vi "SubVI_Files_to_epochs_rev2.vi"(6 "Ch_sel":i32[](array[numeric])=[0, 1, 1, 1, 0], 8 "error in (no error)":errorcluster, 9 "Restrict?":bool, 11 "folder names":string[](array[string])) -> (0 "error out":errorcluster, 1 "Number of Trials":i32, 2 "Rest Epochs":dbl[][](array[numeric]), 3 "Go Epochs":dbl[][](array[numeric]))   [LabVIEW 2020]
uses:
  <vilib>/Analysis/baseanly.llb/Mean (DBL).vi
  <vilib>/Analysis/NI_AALBase.lvlib
panel:
  out "Trial number":i32
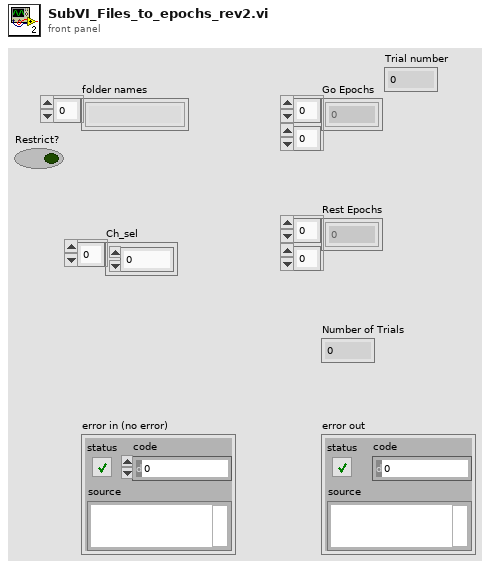
[diagram p1: front panel]
types:
  T1 = enum16{"open", "open or create", "create or replace", "create", "open (read-only)"}
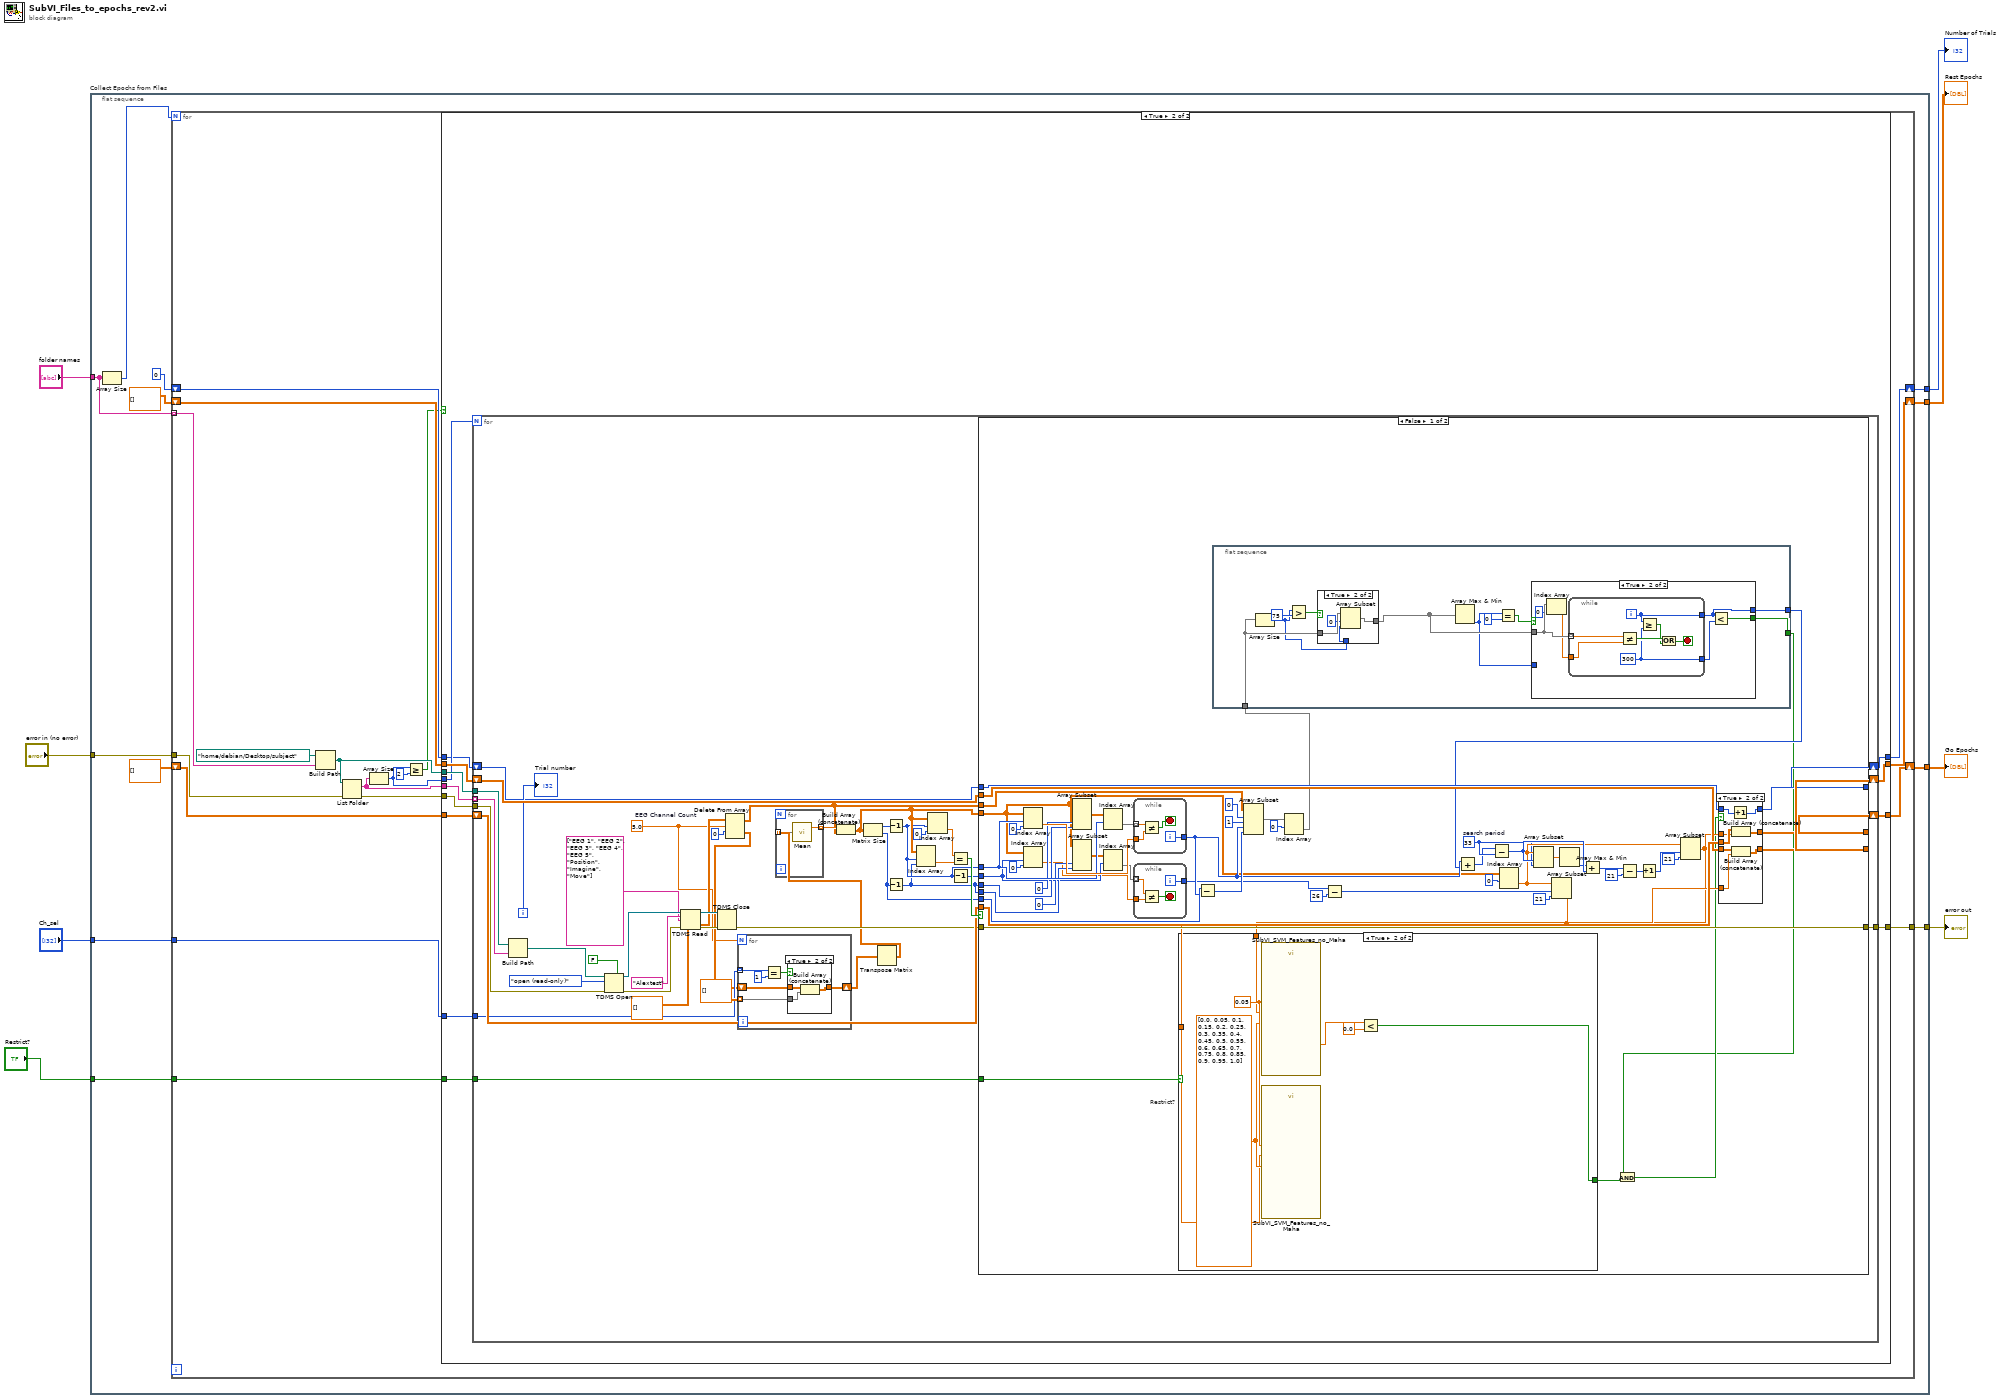
[diagram p0: block diagram]
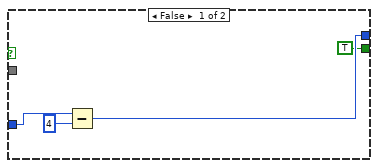
[diagram p4: hidden frame]
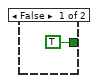
[diagram p6: hidden frame]
diagram:
  n1 = flat-sequence "Collect Epochs from Files" {
    tunnel: "folder names" -> [w19]
    tunnel: "error in (no error)" -> [w18]
    tunnel: [w15] -> w5
    tunnel: [w14] -> w6
    tunnel: [w13] -> w7
    tunnel: [w11] -> w8
    tunnel: "Restrict?" -> [w10]
    tunnel: "Ch_sel" -> [w9]
    frame #0 {
      n2 = Array Size(array=w19) -> (size(s)=w20:i32)
      n3 = for {
        N: w20 -> [_]
        tunnel: w19 -> [w38] mode=indexing
        tunnel: w18 -> [w37]
        tunnel: [w23] -> w13
        shift-right: [w32] -> w15
        shift-left: dbl[][] [] ("Data Buffer") -> [w33]
        shift-right: [w30] -> w14
        shift-left: dbl[][] [] ("Data Buffer") -> [w31]
        shift-right: [w28] -> w11
        shift-left: 0 -> [w29]
        tunnel: w10 -> [w22]
        tunnel: w9 -> [w21]
        n4 = Build Path(base path=path "/home/debian/Desktop/subject", name or relative path=w38) -> (appended path=w34:path)
        n5 = List Folder(path=w34, error in=w37) -> (filenames=w36:string[], error out=w24:errorcluster)  [unwired: 2 in, 2 out]
        n6 = Array Size(array=w36) -> (size(s)=w27:i32)
        n7 = Greater Or Equal?(x=w27, y=2) -> (x >= y?=w25:bool)
        n8 = case shown="True" w25 {
          tunnel: w36 -> [_ w55]
          tunnel: w34 -> [_ w54]
          tunnel: w33 -> [w41 w53]
          tunnel: [w41 w52] -> w32
          tunnel: w31 -> [w40 w51]
          tunnel: [w40 w50] -> w30
          tunnel: w29 -> [w42 w46]
          tunnel: w27 -> [_ w49]
          tunnel: [w42 w45] -> w28
          tunnel: w24 -> [w39 w48]
          tunnel: [w39 w47] -> w23
          tunnel: w22 -> [_ w44]
          tunnel: w21 -> [_ w43]
          frame False {
          }
          frame True {
            n9 = for {
              N: w49 -> [_]
              tunnel: w55 -> [w90] mode=indexing
              tunnel: w54 -> [w91]
              shift-right: [w81] -> w52
              shift-left: w53 -> [w82]
              shift-right: [w83] -> w50
              shift-left: w51 -> [w84]
              tunnel: w48 -> [w74]
              tunnel: [w69] -> w47
              shift-right: [w66] -> w45
              shift-left: w46 -> [w67]
              tunnel: w44 -> [w62]
              tunnel: w43 -> [w58]
              i -> [w68]
              w57 = 5.0  # EEG Channel Count
              n10 = Build Path(base path=w91, name or relative path=w90) -> (appended path=w89:path)
              n11 = TDMS Open(5:FALSE ("create index file? (T)"), 8:w74, 10:T1."open (read-only)" ("operation (0:open)"), 11:w89) -> (0:w95:errorcluster, 3:w93:refnum<k34>)  [unwired: 3 in]
              n12 = TDMS Read(0:w93, 5:"Alextest" ("group name in (Untitled)"), 7:string[] ["EEG 1", "EEG 2", "EEG 3", "EEG 4", "EEG 5", "Position", "Imagine", "Move"] ("channel name(s) in (Untitled)"), 11:w95, 12:dbl[][] [] ("Data Buffer")) -> (4:w92:refnum<k34>, 10:w78:dbl[][], 15:w94:errorcluster)  [unwired: 3 in, 3 out]
              n13 = TDMS Close(8:w94, 11:w92) -> (0:w70:errorcluster)  [unwired: 1 out]
              n14 = Delete From Array(array=w78, length=w57, index (row)=0) -> (deleted portion=w61:dbl[][], array with subset deleted=w72:dbl[][])  [unwired: 1 in]
              n15 = for {
                N: w57 -> [_]
                tunnel: w61 -> [w101] mode=indexing
                tunnel: w58 -> [w104] mode=indexing
                shift-right: [w100] -> w60
                shift-left: dbl[][] [] -> [w99]
                n16 = Equal?(x=w104, y=1) -> (x = y?=w102:bool)
                n17 = case shown="True" w102 {
                  tunnel: w101 -> [_ w108]
                  tunnel: [w105 w107] -> w100
                  tunnel: w99 -> [w105 w106]
                  frame False {
                  }
                  frame True {
                    n18 = Build Array (concatenate)(w106, w108) -> (w107:dbl[][])
                  }
                }
              }
              n19 = Transpose Matrix(1:w60) -> (0:w59:dbl[][])
              n20 = for {
                tunnel: w59 -> [w110] mode=indexing
                tunnel: [w109] -> w76 mode=indexing
                n21 = call-poly <vilib>:"Mean.vi"("X"=w110) -> ("mean"=w109:dbl)  [unwired: 1 out]
              }
              n22 = Build Array (concatenate)(w76, w72) -> (w75:dbl[][])
              n23 = Matrix Size(0:w75) -> (1:w79:i32, 2:w71:i32)
              n24 = Decrement(x=w79) -> (x-1=w65:i32)
              n25 = Decrement(x=w71) -> (x-1=w63:i32)
              n26 = Index Array(array=w75, index (row)=w65, index (col)=w63) -> (element=w86:dbl)
              n27 = Index Array(array=w75, index (row)=w65, index (col)=0 ("disabled index (col)")) -> (element=w87:dbl)
              n28 = Equal?(x=w87, y=w86) -> (x = y?=w85:bool)
              n29 = Decrement(x=w65) -> (x-1=w64:i32)
              n30 = case shown="False" w85 {
                tunnel: w84 -> [w149 w227]
                tunnel: [w148 w227] -> w83
                tunnel: w82 -> [w151 w226]
                tunnel: [w150 w226] -> w81
                tunnel: w75 -> [w129 _]
                tunnel: w65 -> [w146 _]
                tunnel: w63 -> [w144 _]
                tunnel: w72 -> [w141 _]
                tunnel: w71 -> [w140 _]
                tunnel: w70 -> [w133 w225]
                tunnel: [w133 w225] -> w69
                tunnel: w67 -> [w131 w224]
                tunnel: [w130 w224] -> w66
                tunnel: w64 -> [w124 _]
                tunnel: w63 -> [w125 _]
                tunnel: w62 -> [w114 _]
                frame False {
                  w142 = 33  # search period
                  n31 = Index Array(array=w129, index (row)=w146, index (col)=0 ("disabled index (col)")) -> (element=w162:dbl)
                  n32 = Index Array(array=w129, index (row)=w124, index (col)=0 ("disabled index (col)")) -> (element=w122:dbl)
                  n33 = Array Subset(array=w129, index (col)=0 ("index"), length (col)=w144) -> (w147:dbl[][])  [unwired: 2 in]
                  n34 = Array Subset(array=w129, index (col)=0 ("index"), length (col)=w125) -> (w128:dbl[][])  [unwired: 2 in]
                  n35 = Index Array(array=w147, index (row)=w146) -> (element=w164:dbl[])  [unwired: 1 in]
                  n36 = Index Array(array=w128, index (row)=w124) -> (element=w123:dbl[])  [unwired: 1 in]
                  n37 = while {
                    tunnel: w164 -> [w221] mode=indexing
                    tunnel: w162 -> [w222]
                    tunnel: [w220] -> w132
                    i -> [w220]
                    stop <- w223 stop-if-true
                    n38 = Not Equal?(x=w221, y=w222) -> (x != y?=w223:bool)
                  }
                  n39 = while {
                    tunnel: w123 -> [w206] mode=indexing
                    tunnel: w122 -> [w207]
                    tunnel: [w205] -> w121
                    i -> [w205]
                    stop <- w208 stop-if-true
                    n40 = Not Equal?(x=w206, y=w207) -> (x != y?=w208:bool)
                  }
                  n41 = Subtract(x=w140, y=w132) -> (x-y=w139:i32)
                  n42 = flat-sequence {
                    tunnel: w113 -> [w172]
                    tunnel: [w168] -> w111
                    tunnel: [w166] -> w112
                    frame #0 {
                      n43 = Array Size(array=w172) -> (size(s)=w165:i32)
                      n44 = Greater?(x=w165, y=75) -> (0:w173:bool)
                      n45 = case shown="True" w173 {
                        tunnel: w172 -> [w192 w196]
                        tunnel: [w192 w194] -> w169
                        tunnel: w165 -> [_ w193]
                        frame False {
                        }
                        frame True {
                          n46 = Array Subset(array=w196, index=0, length=w193) -> (w194:dbl[])
                        }
                      }
                      n47 = Array Max & Min(array=w169) -> (min index (indices)=w167:i32)  [unwired: 3 out]
                      n48 = Equal?(x=w167, y=0) -> (x = y?=w170:bool)
                      n49 = case shown="True" w170 {
                        tunnel: w169 -> [_ w184]
                        tunnel: [TRUE w180] -> w168
                        tunnel: [w176 w179] -> w166
                        tunnel: w167 -> [w178 _]
                        frame False {
                          n50 = Subtract(x=w178, y=4) -> (x-y=w176:i32)
                        }
                        frame True {
                          n51 = Index Array(array=w184, index=0) -> (element=w182:dbl)
                          n52 = while {
                            tunnel: w184 -> [w191] mode=indexing
                            tunnel: [w188] -> w179
                            tunnel: [w186] -> w181
                            tunnel: w182 -> [w185]
                            i -> [w188]
                            stop <- w187 stop-if-true
                            w186 = 300 ("y")
                            n53 = Not Equal?(x=w191, y=w185) -> (x != y?=w190:bool)
                            n54 = Greater Or Equal?(x=w188, y=w186) -> (x >= y?=w189:bool)
                            n55 = Or(x=w190, y=w189) -> (x .or. y?=w187:bool)
                          }
                          n56 = Less?(x=w179, y=w181) -> (x < y?=w180:bool)
                        }
                      }
                    }
                  }
                  n57 = Array Subset(array=w141, index (row)=0 ("index"), length (row)=1 ("length"), index (col)=w132, length (col)=w139) -> (w137:dbl[][])
                  n58 = Index Array(array=w137, index (row)=0) -> (element=w113:dbl[])  [unwired: 1 in]
                  n59 = Subtract(x=w121, y=26) -> (x-y=w119:i32)
                  n60 = Add(x=w132, y=w112) -> (x+y=w138:i32)
                  n61 = Subtract(x=w138, y=w142) -> (x-y=w159:i32)
                  n62 = Index Array(array=w129, index (row)=0) -> (element=w153:dbl[])  [unwired: 1 in]
                  n63 = Array Subset(array=w153, index=w159, length=w142) -> (w160:dbl[])
                  n64 = Array Subset(array=w153, index=w119, length=21) -> (w118:dbl[])
                  n65 = Array Max & Min(array=w160) -> (min index (indices)=w158:i32)  [unwired: 3 out]
                  n66 = Add(x=w158, y=w159) -> (x+y=w157:i32)
                  n67 = Subtract(x=w157, y=21) -> (x-y=w155:i32)
                  n68 = Increment(x=w155) -> (x+1=w143:i32)
                  n69 = Array Subset(array=w153, index=w143, length=21) -> (w117:dbl[])
                  n70 = case "Restrict?" shown="True" w114 {
                    tunnel: w118 -> [_ w202]
                    tunnel: w117 -> [_ w201]
                    tunnel: [TRUE w198] -> w115
                    frame False {
                    }
                    frame True {
                      w204 = 0.05 ("dt")
                      w203 = dbl[] [0.0, 0.05, 0.1, 0.15, 0.2, 0.25, 0.3, 0.35, 0.4, 0.45, 0.5, 0.55, 0.6, 0.65, 0.7, 0.75, 0.8, 0.85, 0.9, 0.95, 1.0] ("Sliding_window")
                      n71 = call "SubVI_SVM_Features_no_Maha.vi"("dt"=w204, "window_time"=w203, "Sliding_window"=w201) -> ("min value"=w200:dbl)  [unwired: 5 in, 3 out]
                      n72 = call "SubVI_SVM_Features_no_Maha.vi"("dt"=w204, "window_time"=w203, "Sliding_window"=w202) -> ()  [unwired: 5 in, 4 out]
                      n73 = Less?(x=w200, y=0.0) -> (x < y?=w198:bool)
                    }
                  }
                  n74 = And(x=w111, y=w115) -> (x .and. y?=w116:bool)
                  n75 = case shown="True" w116 {
                    tunnel: w151 -> [w211 w219]
                    tunnel: w117 -> [_ w218]
                    tunnel: [w211 w217] -> w150
                    tunnel: w149 -> [w210 w216]
                    tunnel: w118 -> [_ w215]
                    tunnel: [w210 w214] -> w148
                    tunnel: w131 -> [w209 w213]
                    tunnel: [w209 w212] -> w130
                    frame False {
                    }
                    frame True {
                      n76 = Increment(x=w213) -> (x+1=w212:i32)
                      n77 = Build Array (concatenate)(w219, w218) -> (w217:dbl[][])
                      n78 = Build Array (concatenate)(w216, w215) -> (w214:dbl[][])
                    }
                  }
                }
                frame True {
                }
              }
              "Trial number" <- w68
            }
          }
        }
      }
    }
  }
  "Number of Trials" <- w8
  "error out" <- w7
  "Rest Epochs" <- w6
  "Go Epochs" <- w5
